vi "test_Set-Get Protocol Error.vi"(8 "error in (no error)":errorcluster, 11 "TestCase in":refnum<class "Instrument Addon Scripting API Custom Device Unit Tests.lvclass">) -> (0 "error out":errorcluster, 3 "TestCase out":refnum<class "Instrument Addon Scripting API Custom Device Unit Tests.lvclass">)   [LabVIEW 2018, in "Instrument Addon Scripting API Custom Device Unit Tests.lvclass"]
uses:
  Instrument Addon Scripting API Custom Device Unit Tests.lvclass
  Addon/Support Libraries/Protocols.lvlibp/Protocol Parent/Protocol Parent.lvclass
  Instrument Addon Scripting API Test Assets/Instrument Addon Scripting API Test Assets.lvclass
  <vilib>/addons/_JKI Toolkits/VI Tester/TestCase.llb/TestCase.lvclass
  APIs/Scripting API/Instrument Addon Scripting API.lvlib
  C:/Program Files (x86)/National Instruments/LabVIEW 2018/vi.lib/addons/_JKI Toolkits/VI Tester/TestCase.llb/TestCase.lvclass
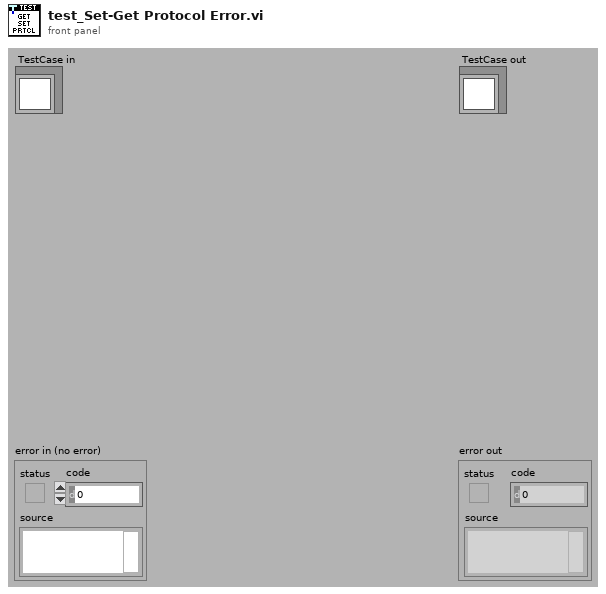
[diagram p1: front panel]
types:
  T1 = typedef "Custom Device API.lvlib/Custom Device Item Ref.ctl" = u64
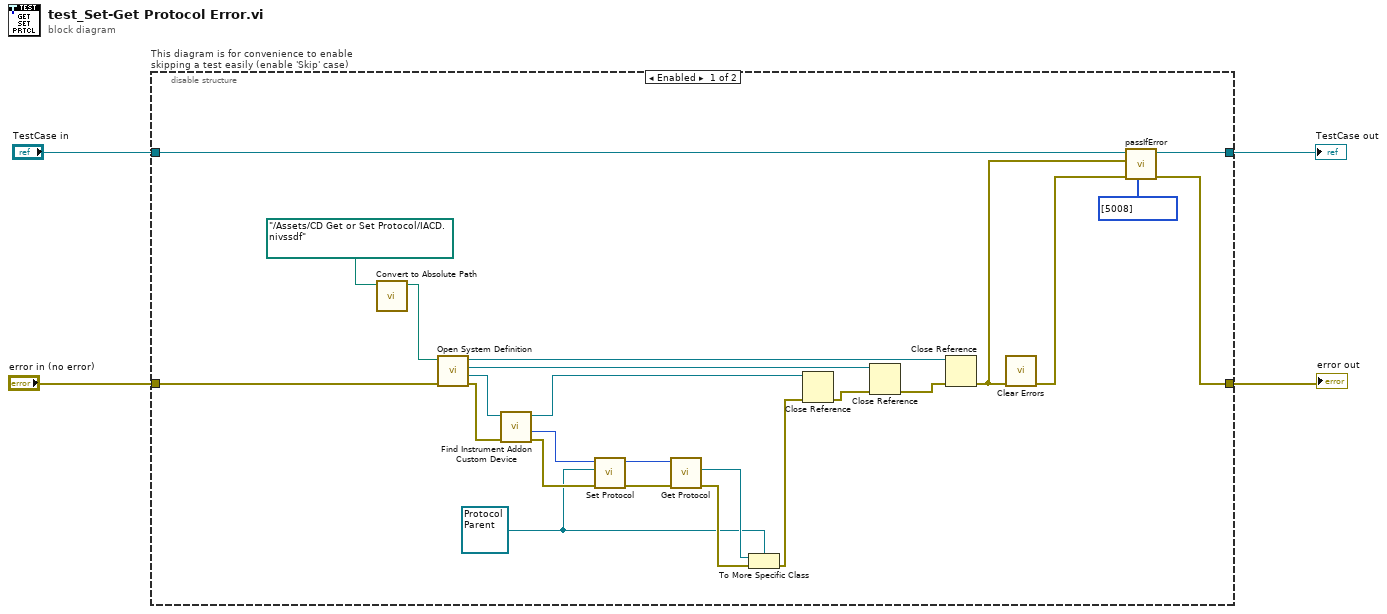
[diagram p0: block diagram]
diagram:
  n1 = disable-structure "This diagram is for convenience to enable skipping a test easily (enable 'Skip' case)" shown="Enabled" {
    disable-tunnel: "TestCase in" -> [w12 w32]
    disable-tunnel: [w11 w30] -> w1
    disable-tunnel: [w7 w31] -> w3
    disable-tunnel: "error in (no error)" -> [w28 w29]
    frame Enabled {
      w13 = refnum<class "Protocol Parent.lvclass"> refnum ("Protocols.lvlibp:Protocol Parent.lvclass")
      n2 = call "Convert to Absolute Path.vi"("System Definition File"=path "../Assets/CD Get or Set Protocol/IACD.nivssdf" ("SDF file")) -> ("Absolute Path"=w26:path)  [unwired: 10 in]
      n3 = call "Open System Definition.vi"("error in (no error)"=w28, "System Definition File"=w26) -> ("error out"=w23:errorcluster, "Target Refnum"=w22:refnum<k24>, "Root Refnum"=w25:refnum<k24>, "System Definition Refnum"=w6:refnum<k24>)  [unwired: 6 in]
      n4 = call "Find Instrument Addon Custom Device.vi"("error in"=w23, "target in"=w22) -> ("error out"=w21:errorcluster, "NodeID"=w20:u64, "target out"=w19:refnum<k24>)  [unwired: 7 in]
      n5 = call "Set Protocol.vi"("Error In"=w21, "Protocol in"=w13, "Instrument Addon Refnum In"=w20) -> ("Error Out"=w17:errorcluster, "Instrument Addon Refnum Out"=w18:T1)  [unwired: 7 in]
      n6 = call "Get Protocol.vi"("Error In"=w17, "Instrument Addon Refnum In"=w18) -> ("Error Out"=w15:errorcluster, "Protocol"=w16:refnum<class "Protocol Parent.lvclass">)  [unwired: 7 in, 1 out]
      n7 = To More Specific Class(target class=w13, reference=w16, error in=w15) -> (error out=w14:errorcluster)  [unwired: 1 out]
      n8 = Close Reference(reference=w19, error in (no error)=w14) -> (error out=w24:errorcluster)
      n9 = Close Reference(reference=w25, error in (no error)=w24) -> (error out=w5:errorcluster)
      n10 = Close Reference(reference=w6, error in (no error)=w5) -> (error out=w9:errorcluster)
      n11 = call <vilib>:"Clear Errors.vi"("error in (no error)"=w9) -> ("error out"=w8:errorcluster)  [unwired: 5 in, 1 out]
      n12 = call-dynamic "passIfError.vi"("passing error codes (default = any error code)"=i32[] [5008], "error in (no error)"=w8, "error"=w9, "TestCase in"=w12) -> ("error out"=w7:errorcluster, "TestCase out"=w11:refnum<class "Instrument Addon Scripting API Custom Device Unit Tests.lvclass">)  [unwired: 6 in]
    }
    frame Disabled {
      # "skip test result while test is under development"
      n13 = call <vilib>:"skip.vi"("error in (no error)"=w29, "TestCase in"=w32) -> ("error out"=w31:errorcluster, "TestCase out"=w30:refnum<class "Instrument Addon Scripting API Custom Device Unit Tests.lvclass">)  [unwired: 8 in]
    }
  }
  "error out" <- w3
  "TestCase out" <- w1
